vi "LeerBD.vi"(8 "error in (no error)":errorcluster) -> (0 "error out":errorcluster, 2 "BD":T1={"NivMaxMenosSens"=97.0, "Incertidumbre"="", "Tol +"="", "Tol -"=""}, 3 "Prueba10 out":refnum<class "Prueba10.lvclass">)   [LabVIEW 2019, in "Prueba10.lvclass"]
uses:
  Prueba10.lvclass
  BD.ctl
  Base de Datos/SQLiteConnector/SQLiteConnection.lvclass
  Base de Datos/Base de Datos.lvclass
panel:
  in  "Tipo Equipo":enum16{"Sonometro", "Calibrador", "Dosimetro"}(ring)
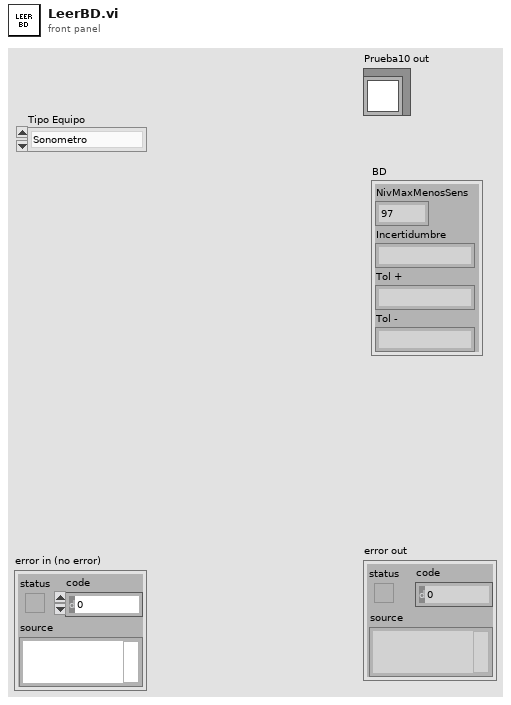
[diagram p1: front panel]
types:
  T1 = typedef "Prueba10.lvclass/BD.ctl" = cluster{"NivMaxMenosSens":dbl, "Incertidumbre":string, "Tol +":string, "Tol -":string}
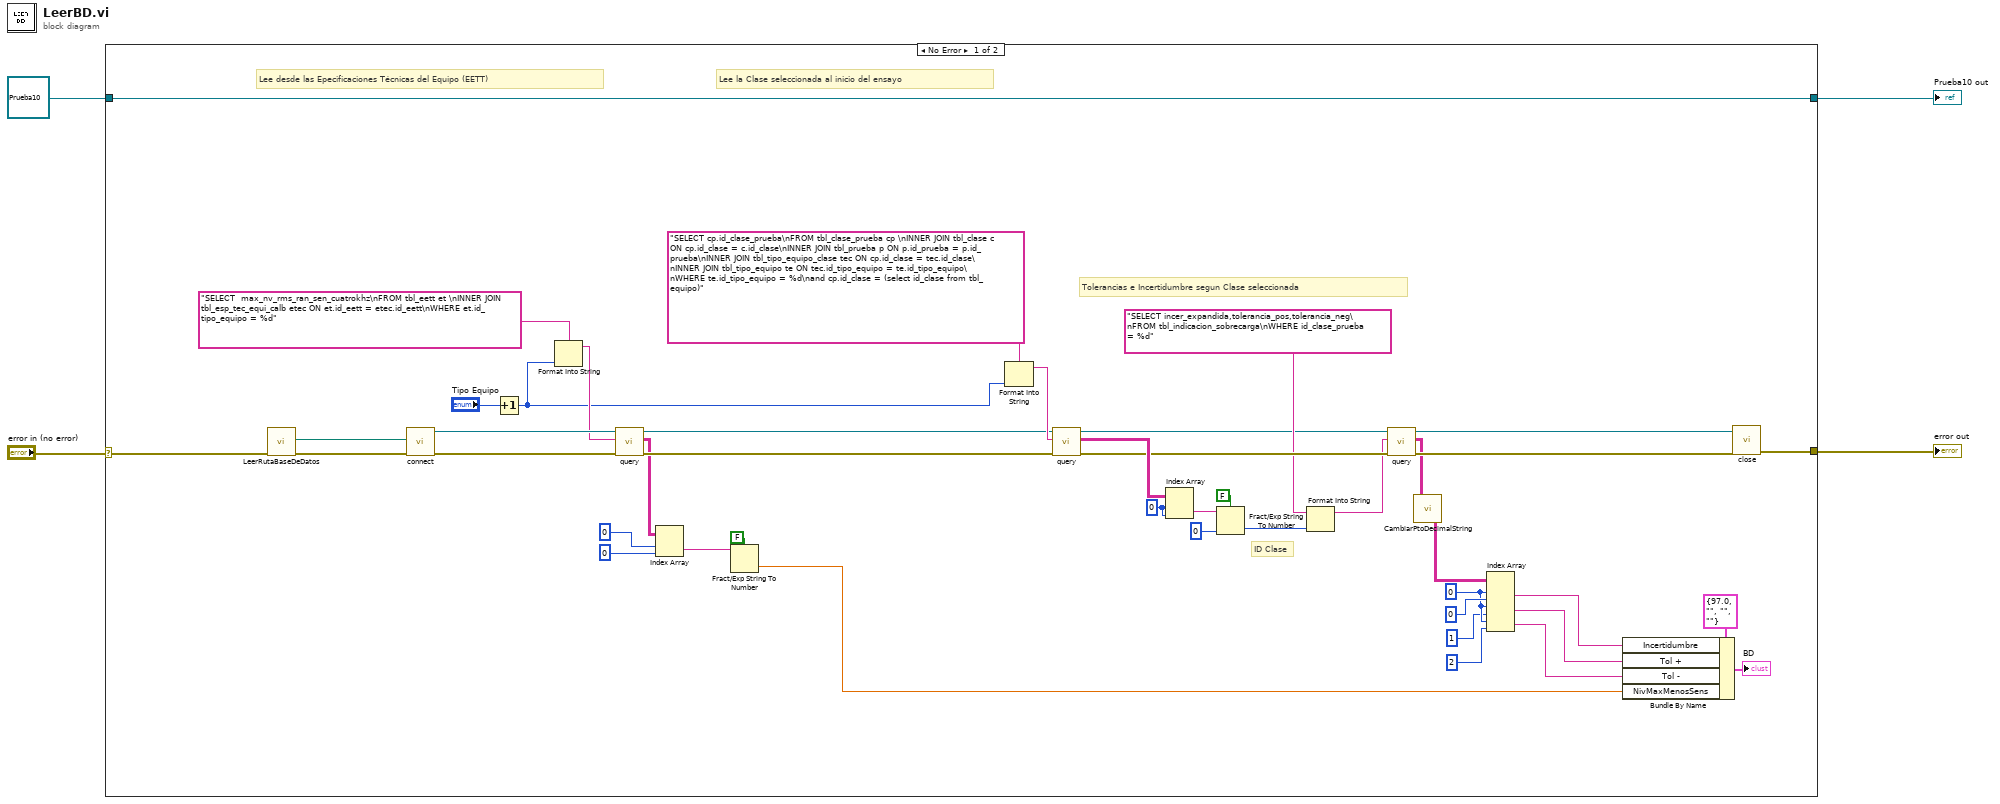
[diagram p0: block diagram]
diagram:
  n1 = case shown="No Error" "error in (no error)" {
    selector: "error in (no error)" -> [w40 w50]
    tunnel: [w26 w50] -> w3
    tunnel: [w48 w49] -> w1
    tunnel: refnum<class "Prueba10.lvclass"> refnum ("Prueba02 in") -> [w48 w49]
    frame No Error {
      w15 = 0 ("index (row)")
      w32 = 0 ("index (row)")
      # "Tolerancias e Incertidumbre segun Clase seleccionada"
      # "ID Clase"
      # "Lee la Clase seleccionada al inicio del ensayo"
      # "Lee desde las Epecificaciones Técnicas del Equipo (EETT)"
      n2 = call "LeerRutaBaseDeDatos.vi"("error in (no error)"=w40) -> ("error out"=w43:errorcluster, "Database Path"=w42:path)  [unwired: 9 in]
      n3 = call "connect.vi"("error in (no error)"=w43, "Database Path"=w42) -> ("error out"=w45:errorcluster, "object out"=w46:refnum<class "SQLiteConnection.lvclass">)  [unwired: 8 in]
      n4 = Increment(x="Tipo Equipo") -> (x+1=w21:enum16{"Sonometro", "Calibrador", "Dosimetro"})
      n5 = Format Into String(format string="SELECT  max_nv_rms_ran_sen_cuatrokhz\nFROM tbl_eett et \nINNER JOIN tbl_esp_tec_equi_calb etec ON et.id_eett = etec.id_eett\nWHERE et.id_tipo_equipo = %d", w21) -> (resulting string=w44:string)  [unwired: 2 in, 1 out]
      n6 = call "query.vi"("error in (no error)"=w45, "SQL Statement"=w44, "object in"=w46) -> ("error out"=w33:errorcluster, "result"=w9:string[][], "object out"=w34:refnum<class "SQLiteConnection.lvclass">)  [unwired: 5 in, 1 out]
      n7 = Index Array(array=w9, index (row)=0, index (col)=0 ("disabled index (col)")) -> (element=w38:string)
      n8 = Fract/Exp String To Number(use system decimal point (T)=FALSE, string=w38) -> (number=w17:dbl)  [unwired: 2 in, 1 out]
      n9 = Format Into String(format string="SELECT cp.id_clase_prueba\nFROM tbl_clase_prueba cp \nINNER JOIN tbl_clase c ON cp.id_clase = c.id_clase\nINNER JOIN tbl_prueba p ON p.id_prueba = p.id_prueba\nINNER JOIN tbl_tipo_equipo_clase tec ON cp.id_clase = tec.id_clase\nINNER JOIN tbl_tipo_equipo te ON tec.id_tipo_equipo = te.id_tipo_equipo\nWHERE te.id_tipo_equipo = %d\nand cp.id_clase = (select id_clase from tbl_equipo)", w21) -> (resulting string=w35:string)  [unwired: 2 in, 1 out]
      n10 = call "query.vi"("error in (no error)"=w33, "SQL Statement"=w35, "object in"=w34) -> ("error out"=w27:errorcluster, "result"=w28:string[][], "object out"=w23:refnum<class "SQLiteConnection.lvclass">)  [unwired: 5 in, 1 out]
      n11 = Index Array(array=w28, index (row)=w32, index (col)=w32) -> (element=w30:string)
      n12 = Fract/Exp String To Number(use system decimal point (T)=FALSE, string=w30, default (0 dbl)=0 ("index (row)")) -> (number=w18:i32)  [unwired: 1 in, 1 out]
      n13 = Format Into String(format string="SELECT incer_expandida,tolerancia_pos,tolerancia_neg\nFROM tbl_indicacion_sobrecarga\nWHERE id_clase_prueba = %d", w18) -> (resulting string=w22:string)  [unwired: 2 in, 1 out]
      n14 = call "query.vi"("error in (no error)"=w27, "SQL Statement"=w22, "object in"=w23) -> ("error out"=w24:errorcluster, "result"=w20:string[][], "object out"=w19:refnum<class "SQLiteConnection.lvclass">)  [unwired: 5 in, 1 out]
      n15 = call "CambiarPtoDecimalString.vi"("result"=w20) -> ("result out"=w5:string[][])
      n16 = Index Array(array=w5, index (row) #1=w15, index (col) #1=0 ("disabled index (col)"), index (row) #2=w15, index (col) #2=1 ("disabled index (col)"), index (row) #3=w15, index (col) #3=2 ("disabled index (col)")) -> (element #1=w12:string, element #2=w11:string, element #3=w10:string)
      n17 = Bundle By Name(cluster=T1 {"NivMaxMenosSens"=97.0, "Incertidumbre"="", "Tol +"="", "Tol -"=""} ("BD"), "Incertidumbre"=w12, "Tol +"=w11, "Tol -"=w10, "NivMaxMenosSens"=w17) -> (→"BD":T1)
      n18 = call-dynamic "close.vi"("error in (no error)"=w24, "object in"=w19) -> ("error out"=w26:errorcluster)  [unwired: 8 in, 1 out]
    }
    frame Error {
    }
  }
  "error out" <- w3
  "Prueba10 out" <- w1
